vi "Combo1.vi"   [LabVIEW 2016, in "Test.lvrbt"]
uses:
  Test.lvrbt
  <vilib>/NXT/Block Support/NXT_InputPort.ctl
  <vilib>/NXT/Hardware/Plugins/Tetrix DC Motor/TetrixDCMotorAddress.ctl
  <vilib>/NXT/Hardware/Plugins/Tetrix 180 deg Servo/Tetrix180ServoAddress.ctl
  <vilib>/NXT/NXTIO Xnodes/NXTIONodeSubVIs/TETRIX IO Move Servos.vi
  <vilib>/NXT/Dual Mode Library/Waits/Wait_Num.vi
  <vilib>/NXT/NXTIO Xnodes/NXTIONodeSubVIs/TETRIX IO Move DC Motors.vi
  <vilib>/NXT/Dual Mode Library/Waits/Wait_EV3_Ultrasonic_Centimeter_Closer.vi
  <vilib>/NXT/NXTIO Xnodes/NXTIONodeSubVIs/TETRIX IO Stop DC Motors.vi
  <vilib>/NXT/Dual Mode Library/Waits/Wait_EV3_Ultrasonic_Centimeters_Further.vi
  <vilib>/NXT/NXTIO Xnodes/AddressXNode/NXTIOAddress.xnode
  <vilib>/NXT/Subs/LVHSConnector.ctl
  <vilib>/NXT/NXTIO Xnodes/NXTIOXNode/NXTIO.xnode
  <vilib>/NXT/LegoClasses/BrickReference/BrickReference.lvclass
types:
  T1 = typedef "NXT_InputPort.ctl" = u32
  T2 = typedef "Tetrix180ServoAddress.ctl" = i32
  T3 = cluster{"Tetrix180Servo":T2, "Tetrix180Servo":T2, "Tetrix180Servo":T2, "Tetrix180Servo":T2, "Tetrix180Servo":T2}
  T4 = typedef "LVHSConnector.ctl" = refnum<class "BrickReference.lvclass">
  T5 = typedef "TetrixDCMotorAddress.ctl" = i32
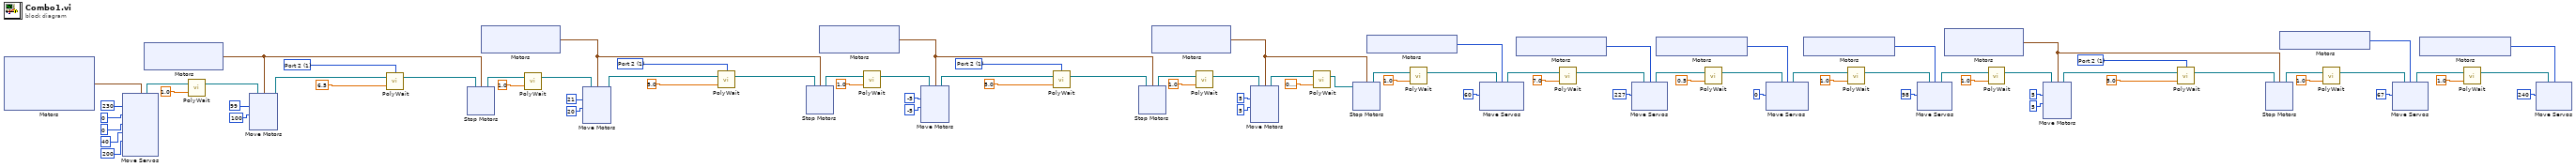
[diagram p0: block diagram]
diagram:
  w21 = T1 1 items=["Port 1", "Port 2", "Port 3", "Port 4"] ("Port (Port 1)")
  w63 = T1 1 items=["Port 1", "Port 2", "Port 3", "Port 4"] ("Port (Port 1)")
  w67 = T1 1 items=["Port 1", "Port 2", "Port 3", "Port 4"] ("Port (Port 1)")
  w68 = T1 1 items=["Port 1", "Port 2", "Port 3", "Port 4"] ("Port (Port 1)")
  n1 = xnode "Motors"() -> ("Motor"=w46:T3)
  n2 = xnode "Move Servos"("Position 5"=u8 200, "Position 4"=u8 40, "Position 3"=u8 0, "Position 2"=u8 0, "Position 1"=u8 230, "Motors"=w46) -> ("NXT/EV3"=w39:T4)  [unwired: 1 in]
  n3 = xnode "Motors"() -> ("Motor"=w80:cluster{"TetrixDCMotor":T5, "TetrixDCMotor":T5})
  n4 = call-poly <vilib>:"PolyWait.vi"("Time (1 sec)"=sgl 1.0, "NXT/EV3"=w39) -> ("NXT/EV3"=w38:T4)  [unwired: 2 in]
  n5 = xnode "Move Motors"("Power/Speed 2"=i8 100, "Power/Speed 1"=i8 99, "Motors"=w80, "NXT/EV3"=w38) -> ("NXT/EV3"=w83:T4)
  n6 = call-poly <vilib>:"PolyWait.vi"("Centimeters (40)"=sgl 6.5, "NXT/EV3"=w83, "Port (Port 1)"=w68) -> ("NXT/EV3"=w81:T4)  [unwired: 1 in]
  n7 = xnode "Stop Motors"("Motors"=w80, "NXT/EV3"=w81) -> ("NXT/EV3"=w79:T4)
  n8 = xnode "Motors"() -> ("Motor"=w71:cluster{"TetrixDCMotor":T5, "TetrixDCMotor":T5})
  n9 = call-poly <vilib>:"PolyWait.vi"("Time (1 sec)"=sgl 1.0, "NXT/EV3"=w79) -> ("NXT/EV3"=w77:T4)  [unwired: 2 in]
  n10 = xnode "Move Motors"("Power/Speed 2"=i8 20, "Power/Speed 1"=i8 21, "Motors"=w71, "NXT/EV3"=w77) -> ("NXT/EV3"=w74:T4)
  n11 = call-poly <vilib>:"PolyWait.vi"("Centimeters (50)"=sgl 5.0, "NXT/EV3"=w74, "Port (Port 1)"=w67) -> ("NXT/EV3"=w72:T4)  [unwired: 1 in]
  n12 = xnode "Stop Motors"("Motors"=w71, "NXT/EV3"=w72) -> ("NXT/EV3"=w69:T4)
  n13 = xnode "Motors"() -> ("Motor"=w27:cluster{"TetrixDCMotor":T5, "TetrixDCMotor":T5})
  n14 = call-poly <vilib>:"PolyWait.vi"("Time (1 sec)"=sgl 1.0, "NXT/EV3"=w69) -> ("NXT/EV3"=w22:T4)  [unwired: 2 in]
  n15 = xnode "Move Motors"("Power/Speed 2"=i8 -5, "Power/Speed 1"=i8 -5, "Motors"=w27, "NXT/EV3"=w22) -> ("NXT/EV3"=w29:T4)
  n16 = call-poly <vilib>:"PolyWait.vi"("Centimeters (40)"=sgl 5.0, "NXT/EV3"=w29, "Port (Port 1)"=w21) -> ("NXT/EV3"=w28:T4)  [unwired: 1 in]
  n17 = xnode "Stop Motors"("Motors"=w27, "NXT/EV3"=w28) -> ("NXT/EV3"=w16:T4)
  n18 = xnode "Motors"() -> ("Motor"=w12:cluster{"TetrixDCMotor":T5, "TetrixDCMotor":T5})
  n19 = call-poly <vilib>:"PolyWait.vi"("Time (1 sec)"=sgl 1.0, "NXT/EV3"=w16) -> ("NXT/EV3"=w17:T4)  [unwired: 2 in]
  n20 = xnode "Move Motors"("Power/Speed 2"=i8 5, "Power/Speed 1"=i8 5, "Motors"=w12, "NXT/EV3"=w17) -> ("NXT/EV3"=w14:T4)
  n21 = call-poly <vilib>:"PolyWait.vi"("Time (1 sec)"=sgl 0.6, "NXT/EV3"=w14) -> ("NXT/EV3"=w11:T4)  [unwired: 2 in]
  n22 = xnode "Stop Motors"("Motors"=w12, "NXT/EV3"=w11) -> ("NXT/EV3"=w13:T4)
  n23 = xnode "Motors"() -> ("Motor"=w58:T2)
  n24 = call-poly <vilib>:"PolyWait.vi"("Time (1 sec)"=sgl 1.0, "NXT/EV3"=w13) -> ("NXT/EV3"=w25:T4)  [unwired: 2 in]
  n25 = xnode "Move Servos"("Position 1"=u8 60, "Motors"=w58, "NXT/EV3"=w25) -> ("NXT/EV3"=w55:T4)
  n26 = xnode "Motors"() -> ("Motor"=w54:T2)
  n27 = call-poly <vilib>:"PolyWait.vi"("Time (1 sec)"=sgl 7.0, "NXT/EV3"=w55) -> ("NXT/EV3"=w52:T4)  [unwired: 2 in]
  n28 = xnode "Move Servos"("Position 1"=u8 227, "Motors"=w54, "NXT/EV3"=w52) -> ("NXT/EV3"=w50:T4)
  n29 = xnode "Motors"() -> ("Motor"=w49:T2)
  n30 = call-poly <vilib>:"PolyWait.vi"("Time (1 sec)"=sgl 0.5, "NXT/EV3"=w50) -> ("NXT/EV3"=w47:T4)  [unwired: 2 in]
  n31 = xnode "Move Servos"("Position 1"=u8 0, "Motors"=w49, "NXT/EV3"=w47) -> ("NXT/EV3"=w36:T4)
  n32 = xnode "Motors"() -> ("Motor"=w34:T2)
  n33 = call-poly <vilib>:"PolyWait.vi"("Time (1 sec)"=sgl 1.0, "NXT/EV3"=w36) -> ("NXT/EV3"=w33:T4)  [unwired: 2 in]
  n34 = xnode "Move Servos"("Position 1"=u8 98, "Motors"=w34, "NXT/EV3"=w33) -> ("NXT/EV3"=w32:T4)
  n35 = xnode "Motors"() -> ("Motor"=w61:cluster{"TetrixDCMotor":T5, "TetrixDCMotor":T5})
  n36 = call-poly <vilib>:"PolyWait.vi"("Time (1 sec)"=sgl 1.0, "NXT/EV3"=w32) -> ("NXT/EV3"=w59:T4)  [unwired: 2 in]
  n37 = xnode "Move Motors"("Power/Speed 2"=i8 5, "Power/Speed 1"=i8 5, "Motors"=w61, "NXT/EV3"=w59) -> ("NXT/EV3"=w64:T4)
  n38 = call-poly <vilib>:"PolyWait.vi"("Centimeters (50)"=sgl 5.0, "NXT/EV3"=w64, "Port (Port 1)"=w63) -> ("NXT/EV3"=w62:T4)  [unwired: 1 in]
  n39 = xnode "Stop Motors"("Motors"=w61, "NXT/EV3"=w62) -> ("NXT/EV3"=w9:T4)
  n40 = xnode "Motors"() -> ("Motor"=w7:T2)
  n41 = call-poly <vilib>:"PolyWait.vi"("Time (1 sec)"=sgl 1.0, "NXT/EV3"=w9) -> ("NXT/EV3"=w6:T4)  [unwired: 2 in]
  n42 = xnode "Move Servos"("Position 1"=u8 67, "Motors"=w7, "NXT/EV3"=w6) -> ("NXT/EV3"=w4:T4)
  n43 = xnode "Motors"() -> ("Motor"=w2:T2)
  n44 = call-poly <vilib>:"PolyWait.vi"("Time (1 sec)"=sgl 1.0, "NXT/EV3"=w4) -> ("NXT/EV3"=w1:T4)  [unwired: 2 in]
  n45 = xnode "Move Servos"("Position 1"=u8 240, "Motors"=w2, "NXT/EV3"=w1) -> ()  [unwired: 1 out]
